vi "Convert Filter to Display String.vi"(11 "Filter Info":T1={"Filter Column"=enum."Description", "Filter Type"=enum."Contains", "Filter Value"="", "New Data?"=FALSE, "Enabled?"=FALSE}) -> (3 "String":string)   [LabVIEW 2020, in "VI Properties Editor.lvlib"]
doc: "Converts <B>Filter Info<B> to a string to be displayed."
uses:
  VI Properties Editor.lvlib
  CTLs/Column Name.ctl
  CTLs/Filter Type.ctl
  CTLs/Filter Info.ctl
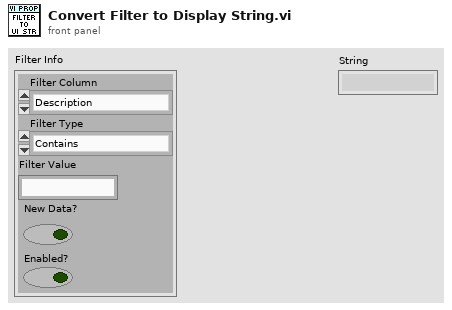
[diagram p1: front panel]
types:
  T1 = typedef "VI Properties Editor.lvlib/Filter Info.ctl" = cluster{"Filter Column":T2, "Filter Type":T3, "Filter Value":string, "New Data?":bool, "Enabled?":bool}
  T2 = typedef "VI Properties Editor.lvlib/Column Name.ctl" = enum16{"Name", "Path", "Type", "Window Title", "Description", "Help Path", "Help Tag", "Custom Title?", "Reentrant?", "Inlined?"}
  T3 = typedef "VI Properties Editor.lvlib/Filter Type.ctl" = enum16{"Contains", "Equals", "Starts with", "Ends with", "Does not contain", "Does not equal", "Is empty", "Is not empty"}
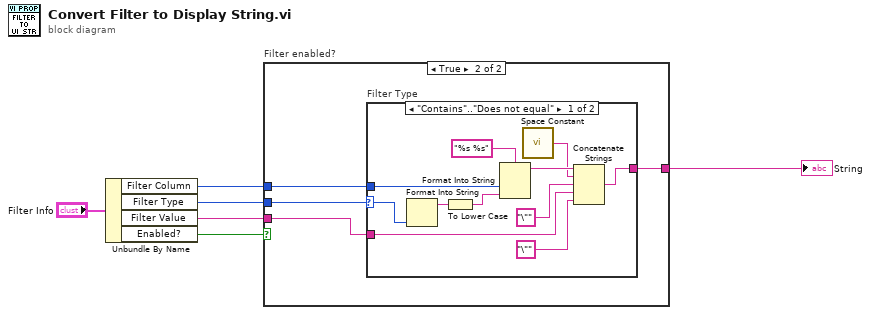
[diagram p0: block diagram]
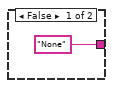
[diagram p2: hidden frame]
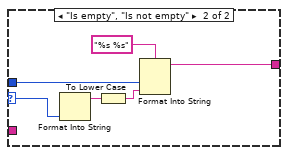
[diagram p3: hidden frame]
diagram:
  n1 = Unbundle By Name("Filter Info") -> ("Filter Column"=w3:T2, "Filter Type"=w5:T3, "Filter Value"=w4:string, "Enabled?"=w2:bool)
  n2 = case "Filter enabled?" shown="True" w2 {
    tunnel: w5 -> [_ w11]
    tunnel: w4 -> [_ w10]
    tunnel: w3 -> [_ w9]
    tunnel: ["None" w8] -> w1
    frame False {
    }
    frame True {
      n3 = case "Filter Type" shown="\"Contains\"..\"Does not equal\"" w11 {
        selector: w11 -> [w19 w25]
        tunnel: w10 -> [w15 _]
        tunnel: w9 -> [w21 w27]
        tunnel: [w12 w26] -> w8
        frame "Contains".."Does not equal" {
          n4 = Format Into String(w19) -> (resulting string=w20:string)  [unwired: 3 in, 1 out]
          n5 = To Lower Case(string=w20) -> (all lower case string=w18:string)
          n6 = Format Into String(format string="%s %s", w21, w18) -> (resulting string=w17:string)  [unwired: 2 in, 1 out]
          n7 = call <vilib>:"Space Constant.vi"() -> ("String"=w16:string)
          n8 = Concatenate Strings(w17, w16, "\"", w15, "\"") -> (w12:string)
        }
        frame "Is empty", "Is not empty" {
          n9 = Format Into String(w25) -> (resulting string=w24:string)  [unwired: 3 in, 1 out]
          n10 = To Lower Case(string=w24) -> (all lower case string=w23:string)
          n11 = Format Into String(format string="%s %s", w27, w23) -> (resulting string=w26:string)  [unwired: 2 in, 1 out]
        }
      }
    }
  }
  "String" <- w1
